vi "MC rep rate.vi"(6 "Timing":T1, 7 "Scan":T2={"Scan Number"=0, "Shot Number"=0, "Scan Data Titles"=[], "ScanData to receive"=[], "Scan Data Array"=[], "Device Names for scan data"=[], "ShotData"=[], "Scans Path"=path "", "scan (T) or noscan"=FALSE, "Scan Info"="", "ScanInfo file path"=path "", "Bin Group"=[], "Scan data"=[], "parameter vals scanned"=[], "tdms file ref"=refnum, "Mcast command"="", "Saved Scans"={"Saved Scans"=[], "Selected Scan"="", "Selected Scan Device"="", "Selected Scan Variable"="", "Current Scan Number"=0, "Total scan number"=0, "Total number of devices"=0, "Total number of shot request"=0, "Current device number"=0, "Current Shot request"=0, "File scan type"=enum."Multi parameter scan", "File scan sections"=[], "bin numbers"=[]}, "dev space var"=[], "reference vi tcp multi read"=refnum, "Scan time elapsed"=0.0, "number BG shots DB"=0, "File Scan Values"=[], "Scan Type"=enum."NoScan", "Scan setup"={"Scan Start"=1.0, "Scan End"=10.0, "Scan Step Size"=1.0, "# Shots Each Step"=10, "single direction?"=TRUE}, "TDMS path"=path "", "QueueDevStatusTCP"=refnum, "TCP subscriptions info"=[], "ShotDataQueuesAndEvents"={"TCPshotDataQueue"=refnum, "TCPShotDataStopQueue"=refnum, "tcp data event"=refnum, "ScanData event reg ref"=refnum}, "scan info popup"=FALSE} {"Scan setup"."Scan Start" format="%#.9p"; "Scan setup"."Scan End" format="%#.9p"; "Scan setup"."Scan Step Size" format="%#.9p"}, 8 "error in (no error)":errorcluster, 9 "enable rep rate":bool=TRUE, 10 "Rate (Hz)":dbl=2.0 format="%.2f", 11 "Boolean in":refnum<vi>) -> (0 "error out":errorcluster, 1 "Hz":sgl format="%.2f", 2 "Hz avg":sgl format="%.2f", 3 "Timing 2":T1, 4 "timeout quit scan":bool, 5 "Scan 2":T2={"Scan Number"=0, "Shot Number"=0, "Scan Data Titles"=[], "ScanData to receive"=[], "Scan Data Array"=[], "Device Names for scan data"=[], "ShotData"=[], "Scans Path"=path "", "scan (T) or noscan"=FALSE, "Scan Info"="", "ScanInfo file path"=path "", "Bin Group"=[], "Scan data"=[], "parameter vals scanned"=[], "tdms file ref"=refnum, "Mcast command"="", "Saved Scans"={"Saved Scans"=[], "Selected Scan"="", "Selected Scan Device"="", "Selected Scan Variable"="", "Current Scan Number"=0, "Total scan number"=0, "Total number of devices"=0, "Total number of shot request"=0, "Current device number"=0, "Current Shot request"=0, "File scan type"=enum."Multi parameter scan", "File scan sections"=[], "bin numbers"=[]}, "dev space var"=[], "reference vi tcp multi read"=refnum, "Scan time elapsed"=0.0, "number BG shots DB"=0, "File Scan Values"=[], "Scan Type"=enum."NoScan", "Scan setup"={"Scan Start"=1.0, "Scan End"=10.0, "Scan Step Size"=1.0, "# Shots Each Step"=10, "single direction?"=TRUE}, "TDMS path"=path "", "QueueDevStatusTCP"=refnum, "TCP subscriptions info"=[], "ShotDataQueuesAndEvents"={"TCPshotDataQueue"=refnum, "TCPShotDataStopQueue"=refnum, "tcp data event"=refnum, "ScanData event reg ref"=refnum}, "scan info popup"=FALSE} {"Scan setup"."Scan Start" format="%#.9p"; "Scan setup"."Scan End" format="%#.9p"; "Scan setup"."Scan Step Size" format="%#.9p"})   [LabVIEW 2020]
uses:
  MC scan cluster.ctl
  Scan Tab Enum.ctl
  scan parameters.ctl
  Shared/GUI_Template/TCP subscription info cluster.ctl
  Shared/GUI_Template/GUI_master/tcp_new_data_event.ctl
  Shared/GUI_Template/GUI_master/tcp new data cluster.ctl
  MC timing cluster.ctl
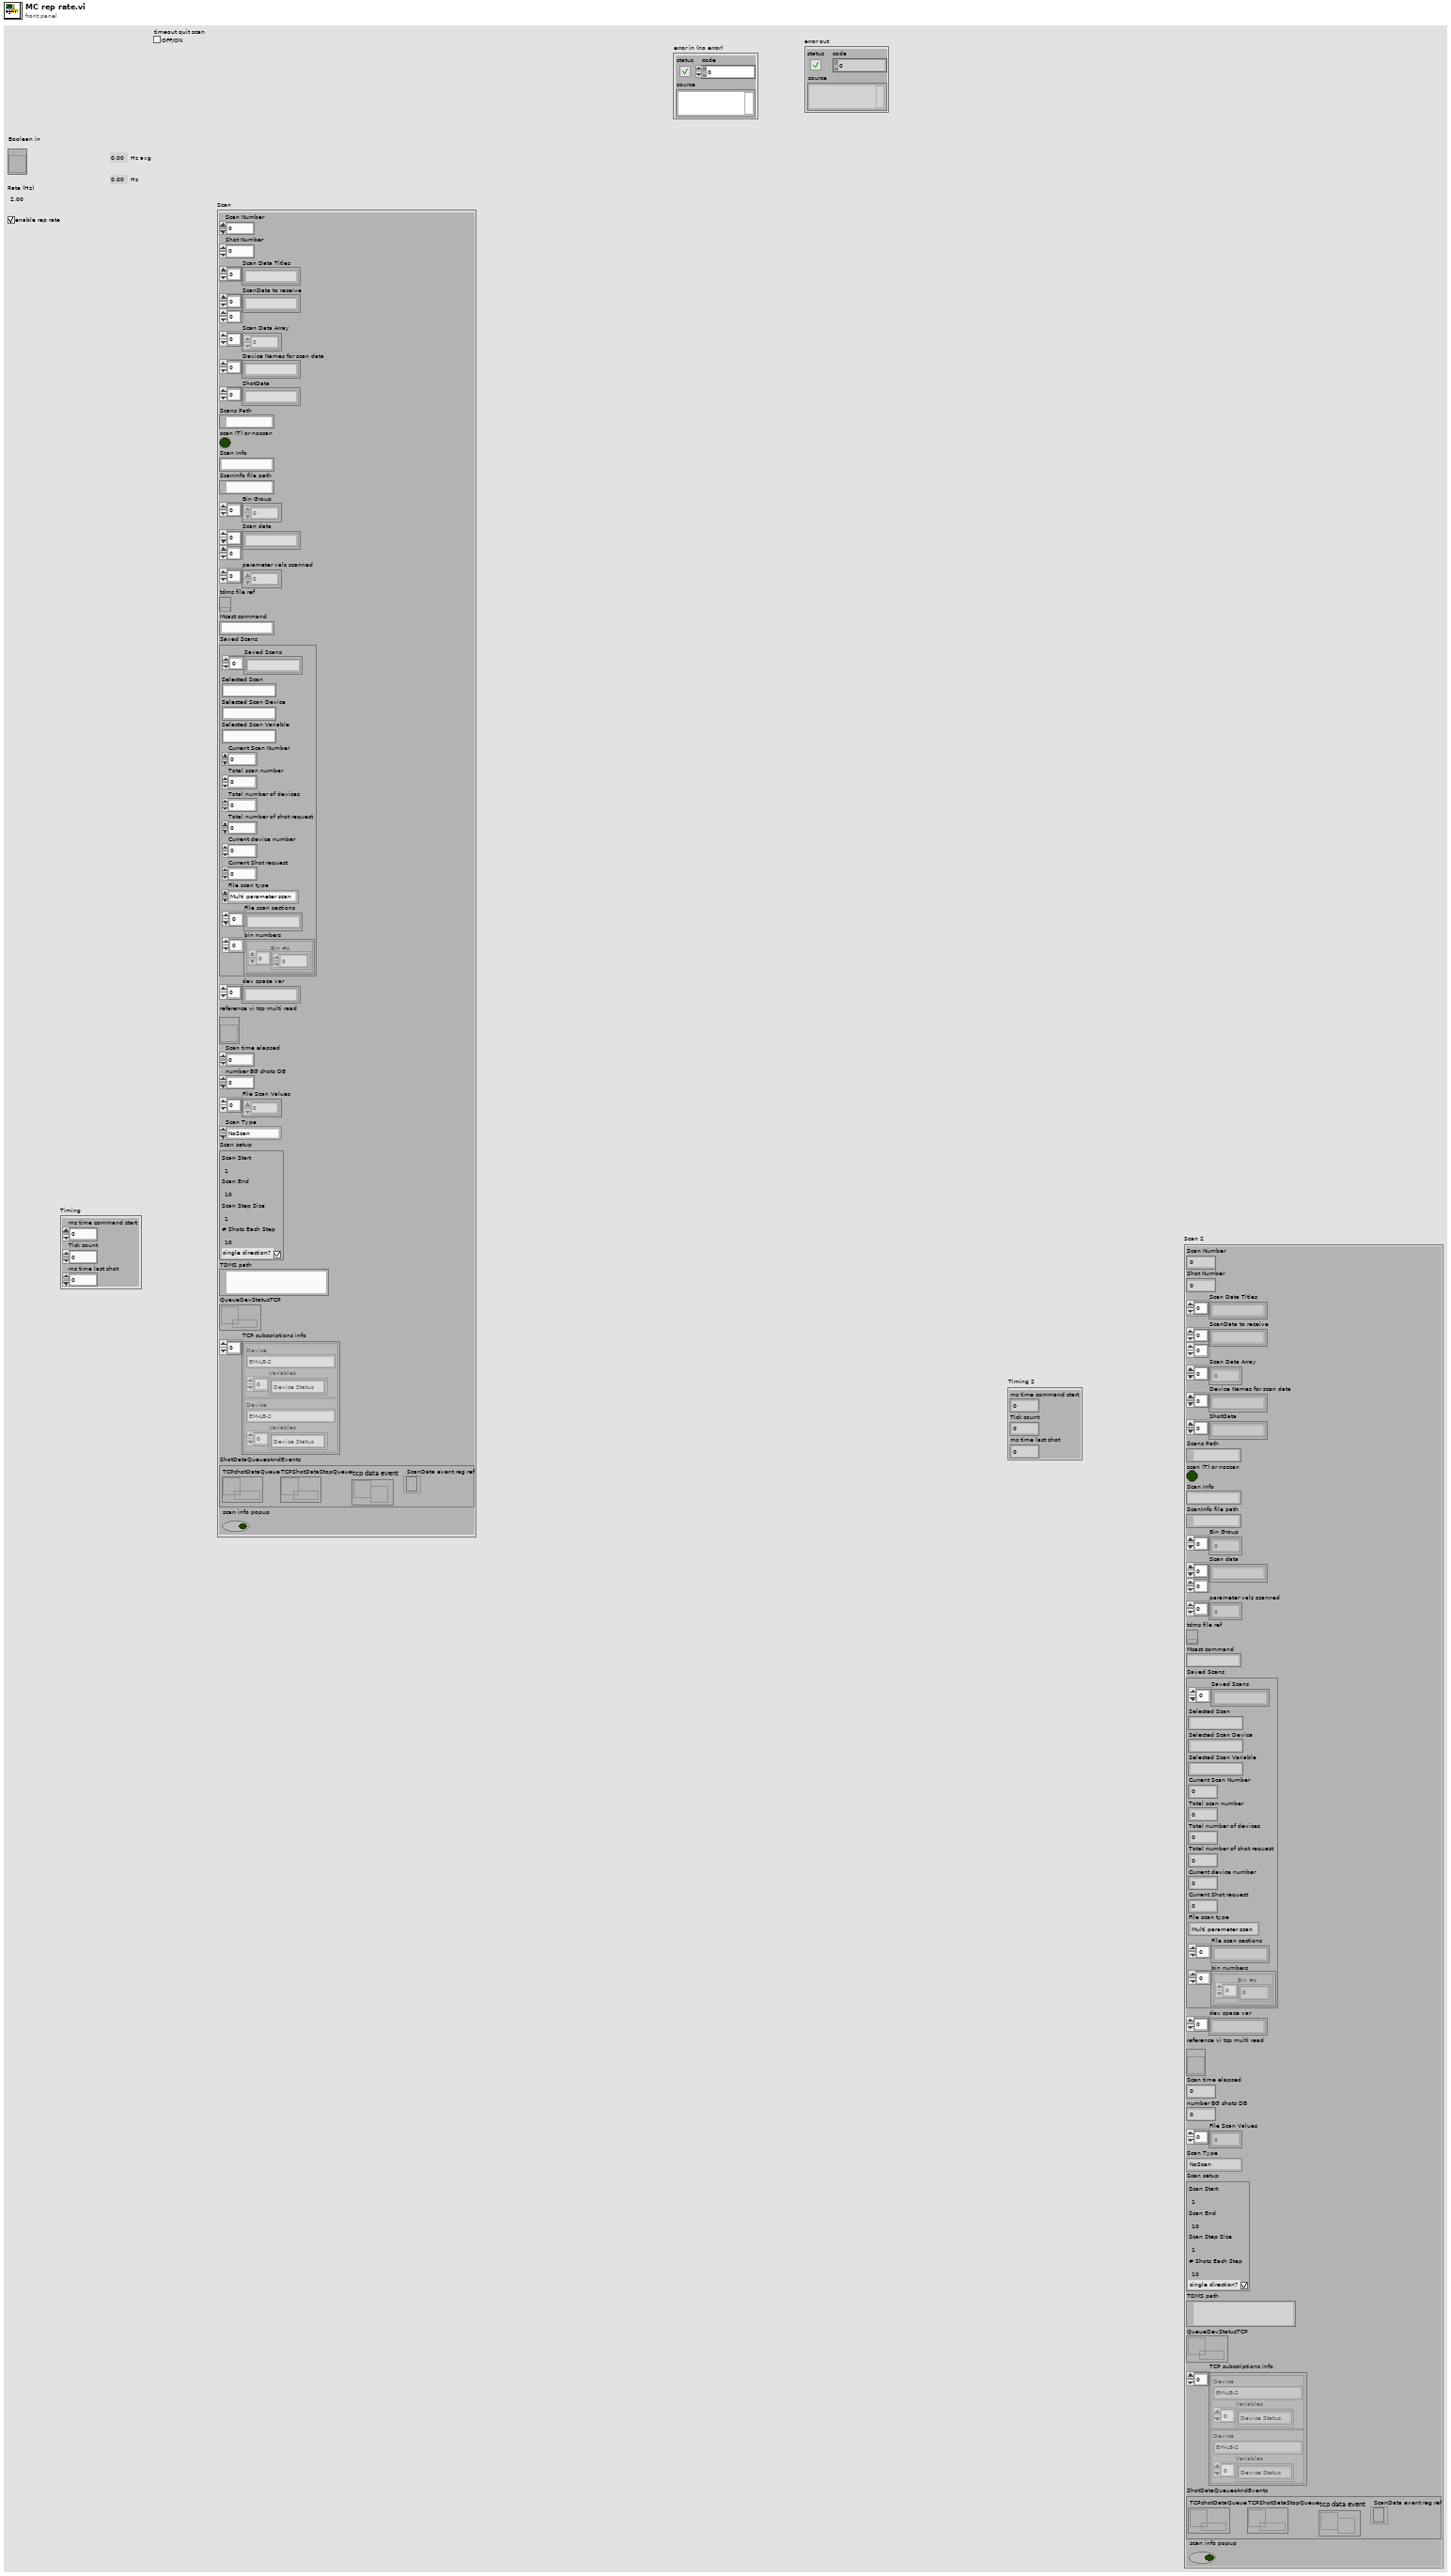
[diagram p1: front panel]
types:
  T1 = typedef "MC timing cluster.ctl" = cluster{"ms time command start":u32, "Tick count":u32, "ms time last shot":u32}
  T2 = typedef "MC scan cluster.ctl" = cluster{"Scan Number":i32, "Shot Number":i32, "Scan Data Titles":string[], "ScanData to receive":string[][], "Scan Data Array":dbl[], "Device Names for scan data":string[], "ShotData":string[], "Scans Path":path, "scan (T) or noscan":bool, "Scan Info":string, "ScanInfo file path":path, "Bin Group":i32[], "Scan data":string[][], "parameter vals scanned":dbl[], "tdms file ref":refnum<k34>, "Mcast command":string, "Saved Scans":cluster{"Saved Scans":string[], "Selected Scan":string, "Selected Scan Device":string, "Selected Scan Variable":string, "Current Scan Number":i32, "Total scan number":i32, "Total number of devices":i32, "Total number of shot request":i32, "Current device number":i32, "Current Shot request":i32, "File scan type":enum32{"Single parameter scan", "Multi parameter scan"}, "File scan sections":string[], "bin numbers":cluster{"Bin #s":i32[]}[]}, "dev space var":string[], "reference vi tcp multi read":refnum<vi>, "Scan time elapsed":sgl, "number BG shots DB":i32, "File Scan Values":dbl[], "Scan Type":T3, "Scan setup":T4, "TDMS path":path, "QueueDevStatusTCP":refnum<queue>, "TCP subscriptions info":T5, "ShotDataQueuesAndEvents":cluster{"TCPshotDataQueue":refnum<queue>, "TCPShotDataStopQueue":refnum<queue>, "tcp data event":T6, "ScanData event reg ref":refnum<event-registration>}, "scan info popup":bool}
  T3 = typedef "Scan Tab Enum.ctl" = enum32{"Scan", "File Scan", "NoScan", "Saved Scans", "Remote Scan"}
  T4 = typedef "scan parameters.ctl" = cluster{"Scan Start":dbl, "Scan End":dbl, "Scan Step Size":dbl, "# Shots Each Step":u32, "single direction?":bool}
  T5 = typedef "TCP subscription info cluster.ctl" = cluster{"Device":string, "Variables":string[]}[]
  T6 = typedef "tcp_new_data_event.ctl" = refnum<user-event>
  T7 = typedef "general button2.ctl" = bool
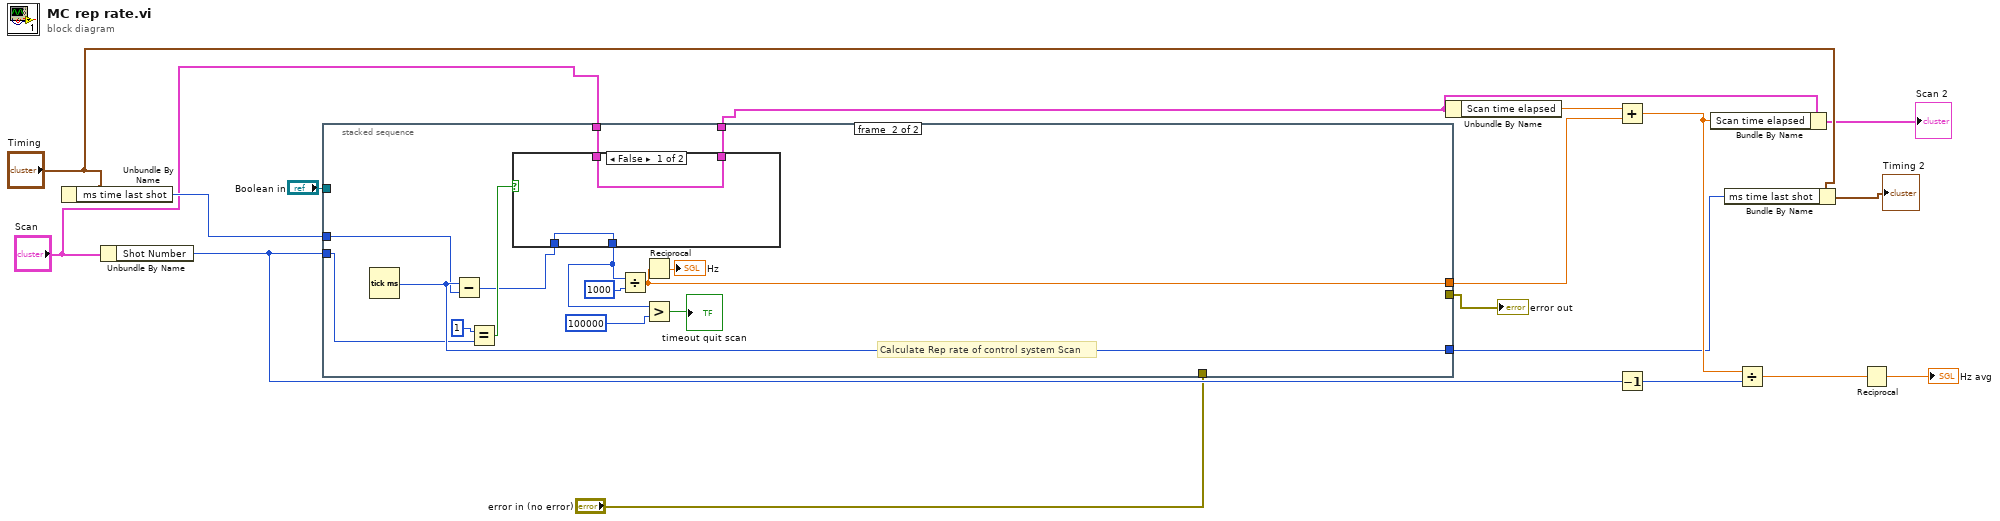
[diagram p0: block diagram]
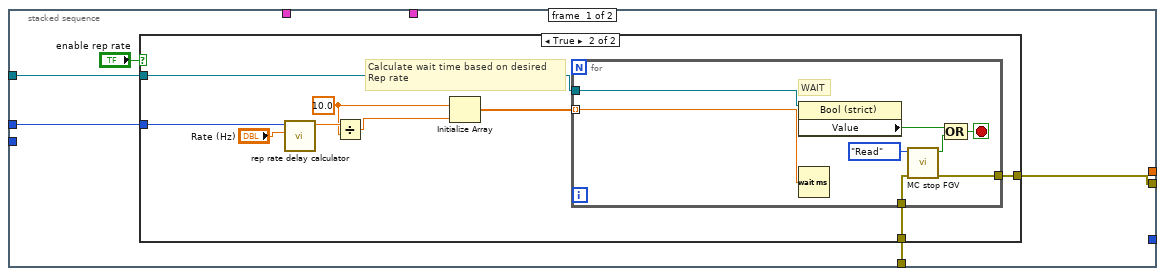
[diagram p2: hidden frame]
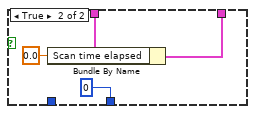
[diagram p4: hidden frame]
diagram:
  n1 = Unbundle By Name("Timing") -> ("ms time last shot"=w7:u32)
  n2 = Unbundle By Name("Scan") -> ("Shot Number"=w11:i32)
  n3 = stacked-sequence {
    tunnel: [_ w51] -> w4
    tunnel: [w22 _] -> w8
    tunnel: w7 -> [w21 w50]
    tunnel: [_ w49] -> w17
    tunnel: w11 -> [_ w47]
    tunnel: "Boolean in" -> [w19 _]
    tunnel: "Scan" -> [_ w45]
    tunnel: [_ w44] -> w5
    tunnel: "error in (no error)" -> [w18 _]
    frame #0 {
      n4 = case shown="True" "enable rep rate" {
        tunnel: [_ w26] -> w22
        tunnel: w21 -> [_ w25]
        tunnel: w19 -> [_ w24]
        tunnel: w18 -> [_ w23]
        frame False {
        }
        frame True {
          w29 = 10.0 ("y")
          # "Calculate wait time based on desired \nRep rate"
          n5 = call "rep rate delay calculator.vi"("max rep rate (Hz)"="Rate (Hz)", "previous shot ms timer value"=w25) -> ("required delay (ms)"=w30:dbl)  [unwired: 8 in, 1 out]
          n6 = Divide(x=w30, y=w29) -> (x/y=w28:dbl)
          n7 = Initialize Array(w29, w28) -> (w27:dbl[])
          n8 = for {
            tunnel: w27 -> [w35] mode=indexing
            tunnel: [w34] -> w26
            tunnel: w24 -> [w33]
            tunnel: w23 -> [w32]
            stop <- w36 stop-if-true
            # "WAIT"
            n9 = property class="Bool (strict)"(reference=w33) -> ("Value"=w38:T7)  [unwired: 1 in, 2 out]
            n10 = Wait (ms)(milliseconds to wait=w35) -> ()  [unwired: 1 out]
            n11 = call "MC stop FGV.vi"("error in"=w32, "Function"=enum16{"Read", "Write", "Clear"}."Read") -> ("error out"=w34:errorcluster, "Stop out"=w37:bool)  [unwired: 8 in]
            n12 = Compound Arithmetic op=OR(w38, w37) -> (w36:T7)
          }
        }
      }
    }
    frame #1 {
      # "Calculate Rep rate of control system Scan"
      n13 = Tick Count (ms)() -> (millisecond timer value=w51:u32)
      n14 = Subtract(x=w51, y=w50) -> (x-y=w43:u32)
      n15 = Equal?(x=1, y=w47) -> (x = y?=w46:bool)
      n16 = case shown="False" w46 {
        tunnel: w45 -> [w55 w59]
        tunnel: [w55 w58] -> w44
        tunnel: [w54 u32 0 ("t")] -> w41
        tunnel: w43 -> [w54 _]
        frame False {
        }
        frame True {
          n17 = Bundle By Name(cluster=w59, "Scan time elapsed"=sgl 0.0 ("Scan.Scan time elapsed")) -> (w58:T2)
        }
      }
      n18 = Divide(x=w41, y=u32 1000) -> (x/y=w49:dbl)
      n19 = Reciprocal(x=w49) -> (1/x=→"Hz":dbl)
      n20 = Greater?(x=w41, y=u32 100000 ("x-y")) -> (0:→"timeout quit scan":bool)
    }
  }
  "error out" <- w8
  n21 = Unbundle By Name(w5) -> ("Scan time elapsed"=w16:sgl)
  n22 = Add(x=w16, y=w17) -> (x+y=w13:dbl)
  n23 = Decrement(x=w11) -> (x-1=w12:i32)
  n24 = Bundle By Name(cluster=w5, "Scan time elapsed"=w13) -> (→"Scan 2":T2)
  n25 = Bundle By Name(cluster="Timing", "ms time last shot"=w4) -> (→"Timing 2":T1)
  n26 = Divide(x=w13, y=w12) -> (x/y=w15:dbl)
  n27 = Reciprocal(x=w15) -> (1/x=→"Hz avg":dbl)
